vi "MergePair.vi"(8 "Sort VI":T1, 10 "B":refnum<data-value>, 11 "A":refnum<data-value>) -> (3 "Merged":refnum<data-value>[](array[refnum]))   [LabVIEW 2020, in "OOPanel.lvlib" / "ArrayManager.lvclass"]
uses:
  <vilib>/IlluminatedG/IG OOPanel/OOPanel/ArrayManager/ArrayManager.lvclass
  <vilib>/IlluminatedG/IG OOPanel/OOPanel/ArrayManager/ArrayManager.lvclass/ArrayManager.ctl
  <vilib>/IlluminatedG/IG OOPanel/OOPanel/ArrayPanel/ArrayPanel.lvclass
  C:/dev/IlluminatedG/.lv-oopanel/OOPanel/Panel/Panel.lvclass
  <vilib>/IlluminatedG/IG OOPanel/OOPanel/ArrayManager/Sort VI Type.ctl
  <vilib>/IlluminatedG/IG OOPanel/OOPanel/Panel/Panel.lvclass
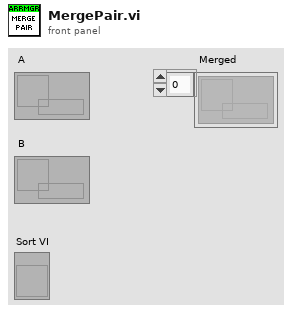
[diagram p1: front panel]
types:
  T1 = typedef "OOPanel.lvlib/ArrayManager.lvclass/Sort VI Type.ctl" = refnum<vi>
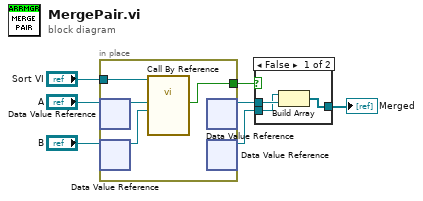
[diagram p0: block diagram]
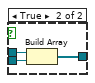
[diagram p2: hidden frame]
diagram:
  n1 = in-place {
    in-place-border: "Sort VI" -> [w11]
    in-place-border: [w8] -> w2
    n2 = in-place-dvr #1("A") -> (w10:refnum<class "ArrayPanel.lvclass">)  [unwired: 1 out]
    n3 = in-place-dvr #2("B") -> (w9:refnum<class "ArrayPanel.lvclass">)  [unwired: 1 out]
    n4 = call-by-ref "?"(reference=w11, "Panel B"=w9, "Panel A"=w10) -> ("A < B"=w8:bool)  [unwired: 10 in, 2 out]
    n5 = in-place-dvr #1() -> (w4:refnum<data-value>)  [unwired: 1 in, 1 out]
    n6 = in-place-dvr #2() -> (w3:refnum<data-value>)  [unwired: 1 in, 1 out]
  }
  n7 = case shown="False" w2 {
    tunnel: w4 -> [w13 w17]
    tunnel: w3 -> [w12 w16]
    tunnel: [w14 w15] -> w1
    frame False {
      n8 = Build Array(w12, w13) -> (w14:refnum<data-value>[])
    }
    frame True {
      n9 = Build Array(w17, w16) -> (w15:refnum<data-value>[])
    }
  }
  "Merged" <- w1
